vi "LVFunction_Imop_SlopesCompute_ModalZonalWavefrontFromCoef.vi"(0 "HasoSlopes":refnum<class "HasoSlopes.lvclass">, 1 "ComputePhaseSet":refnum<class "ComputePhaseSet.lvclass">, 5 "ModalCoef":refnum<class "ModalCoef.lvclass">, 7 "ResidualHasoSlopes":refnum<class "HasoSlopes.lvclass">, 9 "Phase":refnum<class "Phase.lvclass">, 11 "error IO":errorcluster) -> (4 "HasoSlopes (dup)":refnum<class "HasoSlopes.lvclass">, 6 "ModalCoef (dup)":refnum<class "ModalCoef.lvclass">, 8 "ResidualHasoSlopes (dup)":refnum<class "HasoSlopes.lvclass">, 10 "Phase":refnum<class "Phase.lvclass">, 15 "error IO out":errorcluster)   [LabVIEW 2020]
doc: "Compute phase from modal coefficients stored in ModalCoeffs given the\npreferences provided by ComputePhaseSet and adds the residual phase computed\non input HasoSlopes using the modal + zonal reconstruction. Modal coeffs must\nhave a projection pupil set in their preferences.\n\n<B>ComputePhaseSetIn</B> : ComputePhaseSet object.\n<B>ComputePhaseSetOut</B> : ComputePhaseSet object.\n<B>ResidualHasoSlopes</B> : HasoSlopes object containing the input zonal residual slopes.\n<B>ModalCoeffs</B> : ModalCoef object.\n<B>NewResidualHasoSlopes</B> : HasoSlopes object containing the recomputed residual slopes.\n<B>Phase</B> : phase object."
uses:
  ModalCoef.lvclass
  ComputePhaseSet.lvclass
  HasoSlopes.lvclass
  Phase.lvclass
  LVClass_HasoSlopes Read HasoSlopes _ property.vi
  LVClass_ComputePhaseSet Read ComputePhaseSet.vi
  LVClass_ModalCoef Read ModalCoef.vi
  LVClasse_Phase Read SurfaceFloatWithPupil.vi
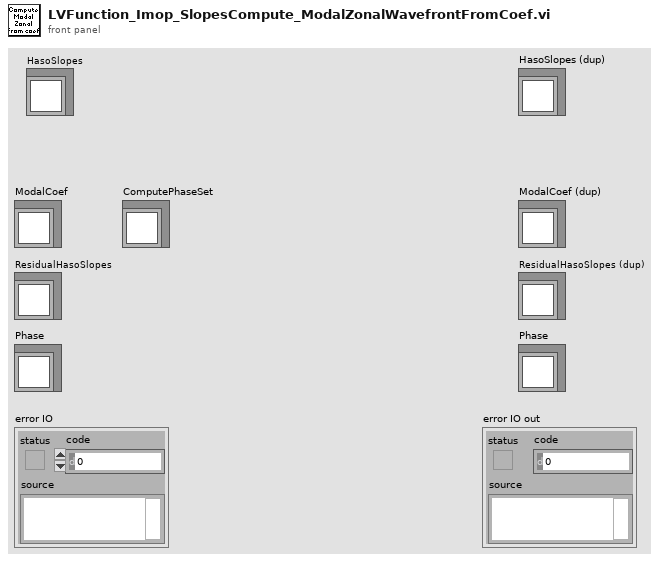
[diagram p1: front panel]
types:
  T1 = typedef "ClassID.ctl" = i64
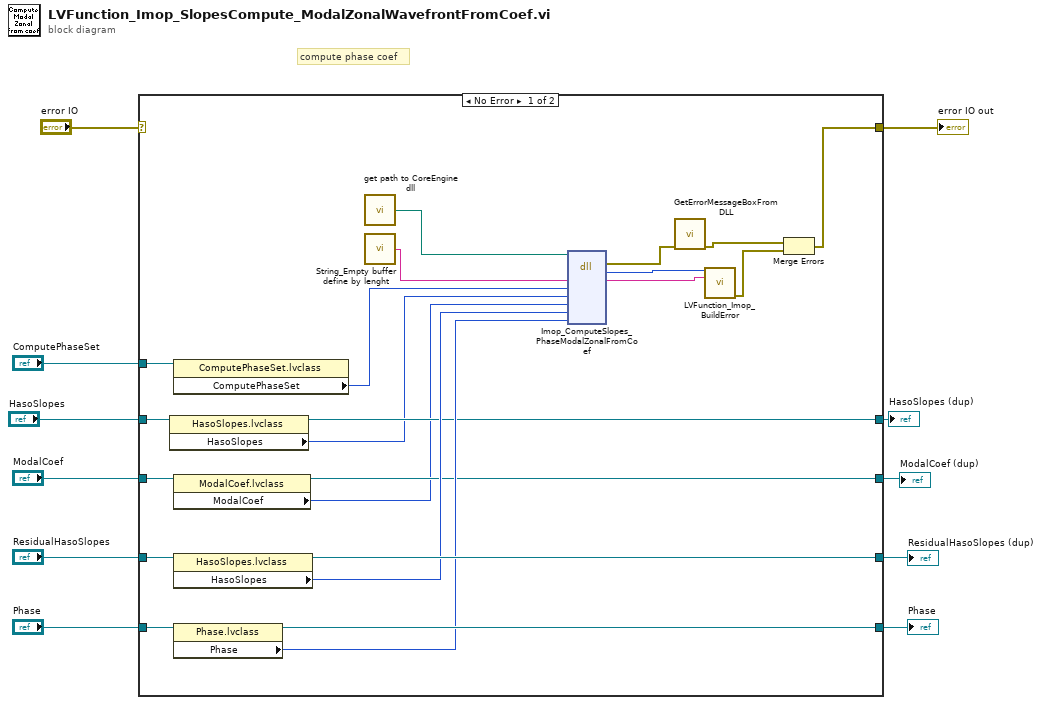
[diagram p0: block diagram]
diagram:
  # "compute phase coef"
  n1 = case shown="No Error" "error IO" {
    selector: "error IO" -> [_ w38]
    tunnel: [w22 w38] -> w10
    tunnel: [w28 w37] -> w5
    tunnel: "Phase" -> [w27 w37]
    tunnel: "ModalCoef" -> [w26 w35]
    tunnel: "ComputePhaseSet" -> [w25 _]
    tunnel: "HasoSlopes" -> [w21 w34]
    tunnel: "ResidualHasoSlopes" -> [w20 w36]
    tunnel: [w18 w36] -> w4
    tunnel: [w15 w35] -> w2
    tunnel: [w14 w34] -> w1
    frame No Error {
      n2 = property class="HasoSlopes.lvclass"(reference=w21) -> (reference out=w14:refnum<class "HasoSlopes.lvclass">, "HasoSlopes"=w13:T1)  [unwired: 1 in, 1 out]
      n3 = property class="ComputePhaseSet.lvclass"(reference=w25) -> ("ComputePhaseSet"=w19:T1)  [unwired: 1 in, 2 out]
      n4 = property class="ModalCoef.lvclass"(reference=w26) -> (reference out=w15:refnum<class "ModalCoef.lvclass">, "ModalCoef"=w12:T1)  [unwired: 1 in, 1 out]
      n5 = property class="HasoSlopes.lvclass"(reference=w20) -> (reference out=w18:refnum<class "HasoSlopes.lvclass">, "HasoSlopes"=w17:T1)  [unwired: 1 in, 1 out]
      n6 = property class="Phase.lvclass"(reference=w27) -> (reference out=w28:refnum<class "Phase.lvclass">, "Phase"=w16:T1)  [unwired: 1 in, 1 out]
      n7 = call "get path to CoreEngine dll.vi"() -> ("path to wavekit library"=w30:path)  [unwired: 14 in, 1 out]
      n8 = call "String_Empty buffer define by lenght.vi"() -> ("Empty buffer"=w31:string)  [unwired: 1 in]
      n9 = dll-call lib="D:/FLE/0.Code/CoreEngine4_Suite/LV2011_interface/DLLs/c_interface_vc100.dll" fn="Imop_ComputeSlopes_PhaseModalZonalFromCoef"(path in=w30, "message"=w31, "ComputePhaseSet"=w19, "ResidualHasoSlopes"=w13, "Modalcoefs"=w12, "NewResidualSlopes"=w17, "Phase"=w16) -> (error out=w29:errorcluster, "return type"=w33:i32, "message"=w32:string)  [unwired: 7 in, 1 out]
      n10 = call "GetErrorMessageBoxFromDLL.vi"("error IN"=w29) -> ("error OUT"=w24:errorcluster)  [unwired: 10 in]
      n11 = call "LVFunction_Imop_BuildError.vi"("code"=w33, "String to Prepend to source (\"\")"=w32) -> ("error out"=w23:errorcluster)  [unwired: 13 in]
      n12 = Merge Errors(w24, w23) -> (w22:errorcluster)
    }
    frame Error {
    }
  }
  "error IO out" <- w10
  "Phase" <- w5
  "ResidualHasoSlopes (dup)" <- w4
  "ModalCoef (dup)" <- w2
  "HasoSlopes (dup)" <- w1
